vi "Create Pattern File Browse.vi"(11 "File Selector Settings":T1(array[cluster])=[{"File Type Selector Label"="ESBR Files", "Array of File Filters"=["BR*.BIN", "BR*.bin"]}, {"File Type Selector Label"="ESBR and ESFI Files", "Array of File Filters"=["BR*.BIN", "BR*.bin", "FI*.BIN", "FI*.bin"]}]) -> (2 "Pattern Label":string="ESBR Files", 3 "Pattern":string)   [LabVIEW 2017]
doc: "This VI will create the <b>Pattern</b> and <b>Pattern Label</b> from the <b>File Selector Settings</b>. This is intended to be used in the Browse VI which will allow multiple file selection types with different patterns."
panel:
  # "#VIA_Ignore Array Default Values"
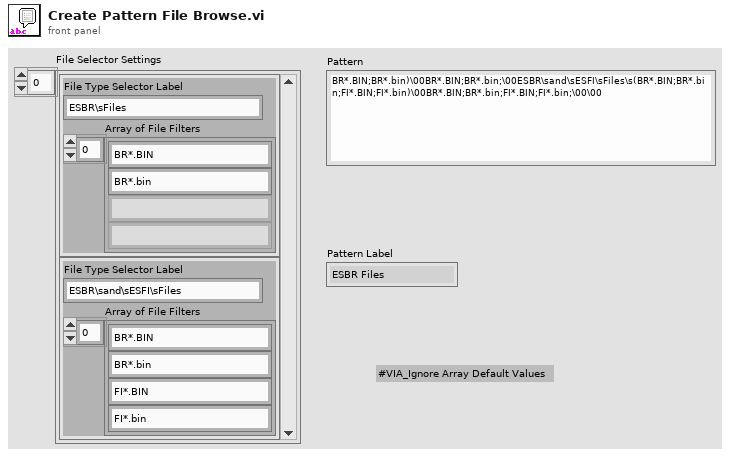
[diagram p1: front panel]
types:
  T1 = cluster{"File Type Selector Label":string, "Array of File Filters":string[]}[]
  T2 = cluster{"File Type Selector Label":string, "Array of File Filters":string[]}
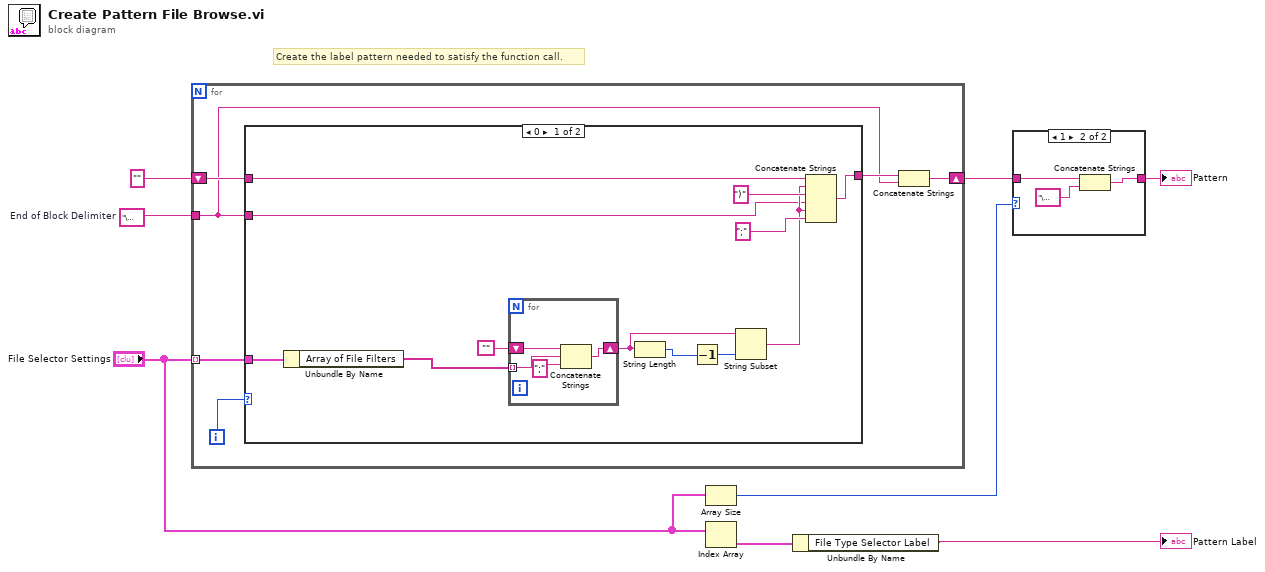
[diagram p0: block diagram]
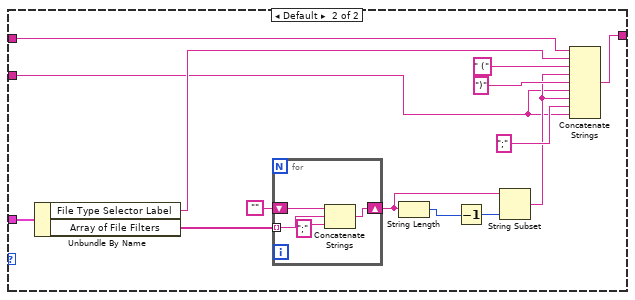
[diagram p3: hidden frame]
diagram:
  w7 = "\u0000"  # End of Block Delimiter
  # "Create the label pattern needed to satisfy the function call."
  n1 = for {
    tunnel: "File Selector Settings" -> [w14] mode=indexing
    shift-right: [w11] -> w2
    shift-left: "" -> [w13]
    tunnel: w7 -> [w10]
    i -> [w9]
    n2 = case shown="0" w9 {
      tunnel: w14 -> [w26 w44]
      tunnel: w13 -> [w17 w32]
      tunnel: [w16 w35] -> w12
      tunnel: w10 -> [w15 w31]
      frame 0 {
        n3 = Unbundle By Name(w26) -> ("Array of File Filters"=w25:string[])
        n4 = for {
          tunnel: w25 -> [w30] mode=indexing
          shift-right: [w28] -> w21
          shift-left: "" -> [w29]
          n5 = Concatenate Strings(w29, w30, ";" ("string")) -> (w28:string)
        }
        n6 = String Length(string=w21) -> (length=w23:i32)
        n7 = Decrement(x=w23) -> (x-1=w22:i32)
        n8 = String Subset(string=w21, length (rest)=w22) -> (substring=w18:string)  [unwired: 1 in]
        n9 = Concatenate Strings(w17, w18, ")" ("string"), w15, w18, ";" ("string")) -> (w16:string)
      }
      frame Default {
        n10 = Unbundle By Name(w44) -> ("File Type Selector Label"=w34:string, "Array of File Filters"=w43:string[])
        n11 = for {
          tunnel: w43 -> [w48] mode=indexing
          shift-right: [w46] -> w39
          shift-left: "" -> [w47]
          n12 = Concatenate Strings(w47, w48, ";" ("string")) -> (w46:string)
        }
        n13 = String Length(string=w39) -> (length=w41:i32)
        n14 = Decrement(x=w41) -> (x-1=w40:i32)
        n15 = String Subset(string=w39, length (rest)=w40) -> (substring=w36:string)  [unwired: 1 in]
        n16 = Concatenate Strings(w32, w34, " (" ("string"), w36, ")" ("string"), w31, w36, ";" ("string"), w31) -> (w35:string)
      }
    }
    n17 = Concatenate Strings(w12, w10) -> (w11:string)
  }
  n18 = Array Size(array="File Selector Settings") -> (size(s)=w3:i32)
  n19 = Index Array(array="File Selector Settings") -> (element=w6:T2)  [unwired: 1 in]
  n20 = Unbundle By Name(w6) -> ("File Type Selector Label"=→"Pattern Label":string)
  n21 = case shown="1" w3 {
    tunnel: w2 -> [w49 w52]
    tunnel: [w49 w51] -> w1
    frame Default {
    }
    frame 1 {
      n22 = Concatenate Strings(w52, "\u0000" ("End of Block Delimiter")) -> (w51:string)
    }
  }
  "Pattern" <- w1
